vi "Autonomous Independent.vi"   [LabVIEW 2018]
doc: "This VI is called when autonomous begins, and will automatically be terminated when autonomous ends. You can carry out timed or sensor driven robot movement independently without needing to return to the caller."
uses:
  <vilib>/Platform/TimedLoop/XDataNode/timing_clust.ctl
  <vilib>/Platform/TimedLoop/XDataNode/nitl_modes.ctl
  <vilib>/Platform/TimedLoop/XDataNode/wakeup.ctl
  Subsystems/Drive/driveCommandEnum.ctl
  Subsystems/HatchPanel/hatchPanelEnum.ctl
  Subsystems/HatchPanel/hatchPanelNotifierCluster.ctl
  <vilib>/Rock Robotics/WPI/DriverStation/WPI_DriverStationDerivedRobotMode.ctl
  Subsystems/Sensors/Limelight/LimelightModeEnum.ctl
  <vilib>/platform/TimedLoop/XDataNode/XDataNode.xnode
  <vilib>/Platform/TimedLoop/XDataNode/XDNodeRunTimeDep.lvlib
panel:
  # "Be sure to right-click and choose Data Operations>>Make Current Value default if you want to save the array values with the VI"
types:
  T1 = typedef "XDNodeRunTimeDep.lvlib/timing_clust.ctl" = cluster{"Expected End [f-1]":u64, "Actual End [f-1]":u64, "Finished Late? [f-1]":bool, "Expected End [i-1]":u64, "Actual End [i-1]":u64, "Finished Late? [i-1]":bool, "Expected Start [i]":u64, "Actual Start [i]":u64, "Expected Start [f]":u64, "Actual Start [f]":u64, "Source Name":string, "Structure Name":string, "Period":i64, "Deadline":i64, "Offset":i64, "Start":i64, "Priority":i32, "Timeout":i32, "Mode":T2, "Wakeup Reason":T3, "Error":errorcluster, "Source Type":string, "Secondary Source Type":string, "Global End Time":u64, "Global Start Time":u64, "Frame Duration":u64, "Iteration Duration":u64, "Assigned CPU":i32, "I/O Scan Engine Mode":u32}
  T2 = typedef "XDNodeRunTimeDep.lvlib/nitl_modes.ctl" = enum32{"No Change", "Process missed periods, maintain original phase", "Discard missed periods, maintain original phase", "Process missed periods, ignore original phase", "Discard missed periods, ignore original phase"}
  T3 = typedef "XDNodeRunTimeDep.lvlib/wakeup.ctl" = enum32{"Normal", "Aborted", "Asynchronous wakeup", "Timing source error", "Timed loop error", "Timeout"}
  T4 = typedef "WPI_MotorControlDeviceRef.ctl" = cluster{"DeviceStatus":errorcluster, "Type":T5, "PWM":cluster{"PWM Channel":T6, "DeadBand":T7}, "CAN":cluster{"Device Number":u8, "SetOutput VI Ref":variant, "GetOutput VI Ref":variant, "Enable VI Ref":variant, "Disable VI Ref":variant, "Data":variant}, "Invert":bool, "DIO PWM":cluster{"PWM \"Enable\" Channel":T6, "DIOChannel":T8, "PWM Rate":dbl}}
  T5 = typedef "WPI_MotorControlType.ctl" = enum16{"PWM", "CAN", "DIO PWM"}
  T6 = typedef "FPGA_DIOPWMChannel.ctl" = enum8{"PWM 0", "PWM 1", "PWM 2", "PWM 3", "PWM 4", "PWM 5", "PWM 6", "PWM 7", "PWM 8", "PWM 9", "PWM MXP 0", "PWM MXP 1", "PWM MXP 2", "PWM MXP 3", "PWM MXP 4", "PWM MXP 5", "PWM MXP 6", "PWM MXP 7", "PWM MXP 8", "PWM MXP 9", "Invalid"}
  T7 = typedef "WPI_PWMDeadband.ctl" = cluster{"Name":string, "maxPositivePwm":i32, "minPositivePwm":i32, "centerPwm":i32, "maxNegativePwm":i32, "minNegativePwm":i32, "angularRange":u16}
  T8 = typedef "FPGA_DIOChannel.ctl" = enum8{"DIO 0", "DIO 1", "DIO 2", "DIO 3", "DIO 4", "DIO 5", "DIO 6", "DIO 7", "DIO 8", "DIO 9", "DIO MXP 0", "DIO MXP 1", "DIO MXP 2", "DIO MXP 3", "DIO MXP 4", "DIO MXP 5", "DIO MXP 6", "DIO MXP 7", "DIO MXP 8", "DIO MXP 9", "DIO MXP 10", "DIO MXP 11", "DIO MXP 12", "DIO MXP 13", "DIO MXP 14", "DIO MXP 15", "SPI Port CS1", "SPI Port CS2", "SPI Port CS3", "SPI Port MISO", "SPI Port MOSI", "Invalid"}
  T9 = typedef "hatchPanelNotifierCluster.ctl" = cluster{"Hatch Panel State":T10, "Mechanism Motion":bool, "Gathering Claw Motion":bool, "Scoring Claw Motion":bool}
  T10 = typedef "hatchPanelEnum.ctl" = enum16{"do nothing", "Stach Mode", "Climb Mode", "Retracted Closed", "Retracted Open", "Extended Closed", "Extended Open"}
  T11 = typedef "driveCommandEnum.ctl" = enum16{"doNothing", "Manuel", "Teleop", "Move to Target", "Climb", "Line Align", "Sonar BrakeTele", "Turn To Angle", "Auto Drive", "Test Auto Forward", "Test Auto Reversed", "Code Drive"}
  T12 = typedef "WPI_DriverStationDerivedRobotMode.ctl" = enum16{"Init", "Execute", "Stop"}
  T13 = typedef "LimelightModeEnum.ctl" = enum16{"SA - Front", "SA - Rear", "SA - Side by Side", "Vision Processing"}
  T14 = cluster{"Hatch Panel State":bool, "Mechanism Motion":bool, "Gathering Claw Motion":bool, "Scoring Claw Motion":bool}
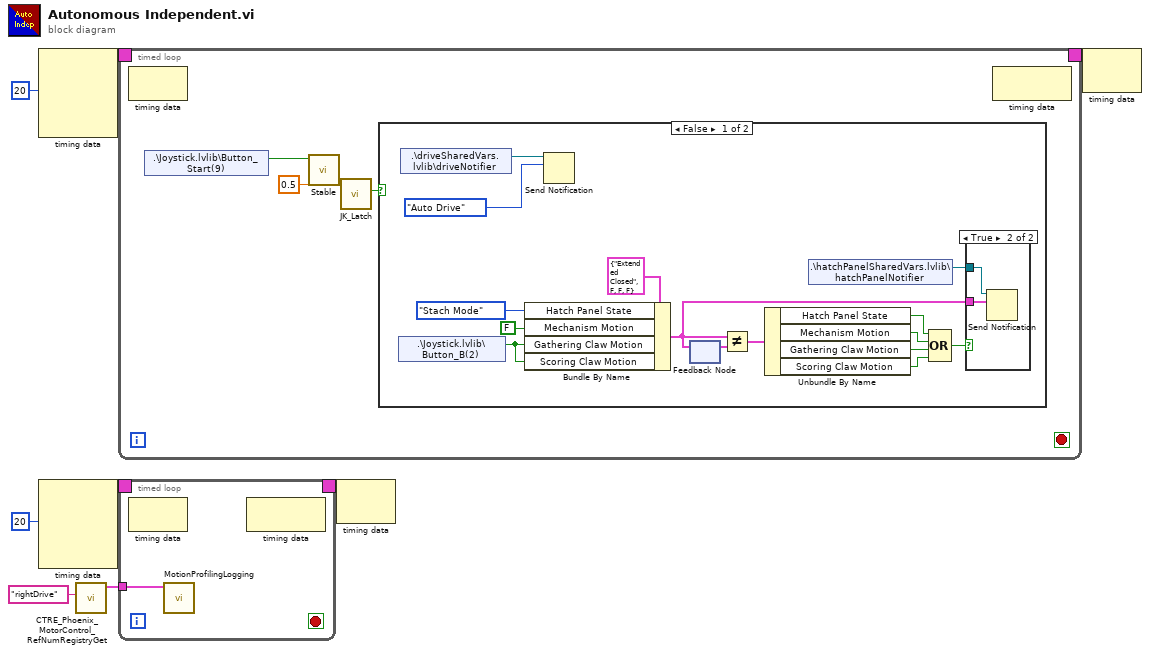
[diagram p0: block diagram]
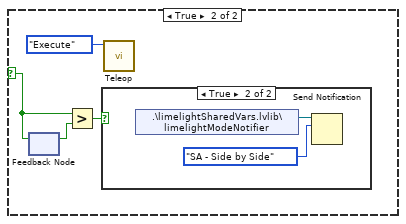
[diagram p3: hidden frame]
diagram:
  n1 = node-c288(i64 20 ("Period")) -> (w8:T1)  [unwired: 3 in]
  n2 = node-c288(i64 20 ("Period")) -> (w4:T1)  [unwired: 3 in]
  n3 = call <vilib>:"CTRE_Phoenix_MotorControl_RefNumRegistryGet.vi"("refnum name"="rightDrive") -> ("PhoenixMotorControlDevRef"=w2:T4)  [unwired: 9 in, 1 out]
  n4 = timed-loop {
    timing: w8 -> [_]
    timing-out: [_] -> w7
    stop <- _ stop-if-true
    n5 = node-c288() -> ()  [unwired: 1 in, 1 out]
    n6 = shared-variable ".\\Joystick.lvlib\\Button_Start(9)"() -> (w12:bool)  [unwired: 1 in, 1 out]
    n7 = call <userlib>:"Stable.vi"("Eval Period (sec)"=0.5, "Signal Input"=w12) -> ("Stable"=w10:bool)  [unwired: 9 in]
    n8 = call <userlib>:"JK_Latch.vi"("Set"=w10) -> ("Q"=w9:bool)  [unwired: 6 in]
    n9 = case shown="False" w9 {
      selector: w9 -> [_ w31]
      frame False {
        n10 = shared-variable ".\\Joystick.lvlib\\Button_B(2)"() -> (w17:bool)  [unwired: 1 in, 1 out]
        n11 = shared-variable ".\\driveSharedVars.lvlib\\driveNotifier"() -> (w27:refnum<notifier>)  [unwired: 1 in, 1 out]
        n12 = Bundle By Name(cluster=T9 {"Hatch Panel State"=enum."Extended Closed", "Mechanism Motion"=FALSE, "Gathering Claw Motion"=FALSE, "Scoring Claw Motion"=FALSE} ("notification"), "Hatch Panel State"=hatchPanelEnum."Stach Mode", "Mechanism Motion"=FALSE, "Gathering Claw Motion"=w17, "Scoring Claw Motion"=w17) -> (w25:T9)
        n13 = Send Notification(notification=driveCommandEnum."Auto Drive", notifier=w27) -> ()  [unwired: 1 in, 2 out]
        n14 = feedback #1() -> (w18:T9)  [unwired: 1 in]
        n15 = feedback-in #1(w25) -> ()
        n16 = Not Equal?(x=w25, y=w18) -> (x != y?=w19:T14)
        n17 = Unbundle By Name(w19) -> ("Hatch Panel State"=w20:bool, "Mechanism Motion"=w21:bool, "Gathering Claw Motion"=w22:bool, "Scoring Claw Motion"=w24:bool)
        n18 = shared-variable ".\\hatchPanelSharedVars.lvlib\\hatchPanelNotifier"() -> (w14:refnum<notifier>)  [unwired: 1 in, 1 out]
        n19 = Compound Arithmetic op=OR(w20, w21, w22, w24) -> (w23:bool)
        n20 = case shown="True" w23 {
          tunnel: w14 -> [_ w29]
          tunnel: w25 -> [_ w28]
          frame False {
          }
          frame True {
            n21 = Send Notification(notification=w28, notifier=w29) -> ()  [unwired: 1 in, 2 out]
          }
        }
      }
      frame True {
        n22 = feedback #2() -> (w32:bool)  [unwired: 1 in]
        n23 = feedback-in #2(w31) -> ()
        n24 = Greater?(x=w31, y=w32) -> (0:w30:bool)
        n25 = case shown="True" w30 {
          frame False {
          }
          frame True {
            n26 = shared-variable ".\\limelightSharedVars.lvlib\\limelightModeNotifier"() -> (w34:refnum<notifier>)  [unwired: 1 in, 1 out]
            n27 = Send Notification(notification=LimelightModeEnum."SA - Side by Side", notifier=w34) -> ()  [unwired: 1 in, 2 out]
          }
        }
        n28 = call "Teleop.vi"("Call Context"=WPI_DriverStationDerivedRobotMode."Execute") -> ()  [unwired: 9 in]
      }
    }
    n29 = node-c288() -> ()  [unwired: 1 in, 1 out]
  }
  n30 = timed-loop {
    timing: w4 -> [_]
    timing-out: [_] -> w3
    tunnel: w2 -> [w38]
    stop <- _ stop-if-true
    n31 = node-c288() -> ()  [unwired: 1 in, 1 out]
    n32 = call "MotionProfilingLogging.vi"("Main Talon"=w38) -> ()  [unwired: 11 in]
    n33 = node-c288() -> ()  [unwired: 1 in, 1 out]
  }
  n34 = node-c288(w3) -> ()  [unwired: 1 out]
  n35 = node-c288(w7) -> ()  [unwired: 1 out]
